vi "SQLGetDiagRec.vi"(4 "error in (no error)":errorcluster, 5 "HandleType":T1(ring)=enum."SQL_HANDLE_ENV", 6 "Status (SQL_SUCCESS=0)":i16, 7 "Input Handle":i32) -> (0 "error out":errorcluster, 3 "Output Handle":i32)   [LabVIEW 2011]
uses:
  Odbc32.dll
panel:
  in  "Boolean":bool
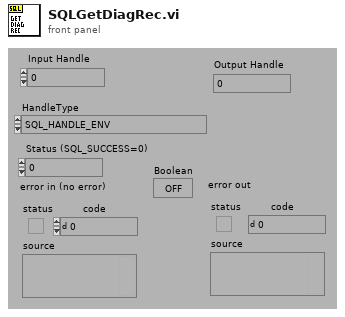
[diagram p1: front panel]
types:
  T1 = enum16{"NOPE", "SQL_HANDLE_ENV", "SQL_HANDLE_DBC", "SQL_HANDLE_STMT", "SQL_HANDLE_DESC"}
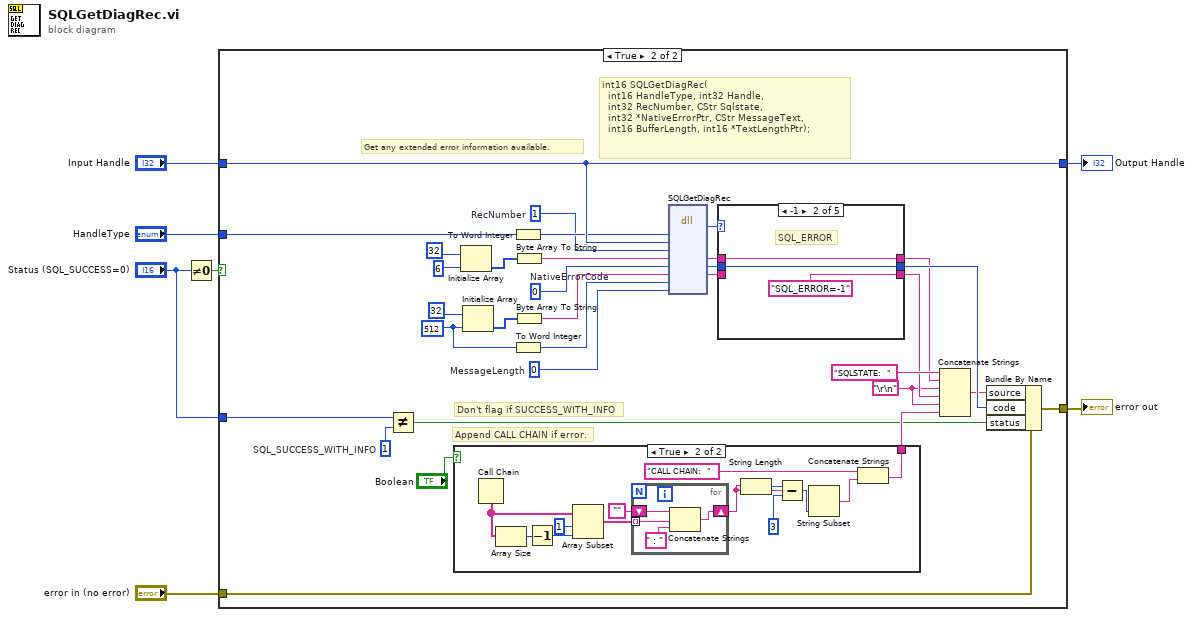
[diagram p0: block diagram]
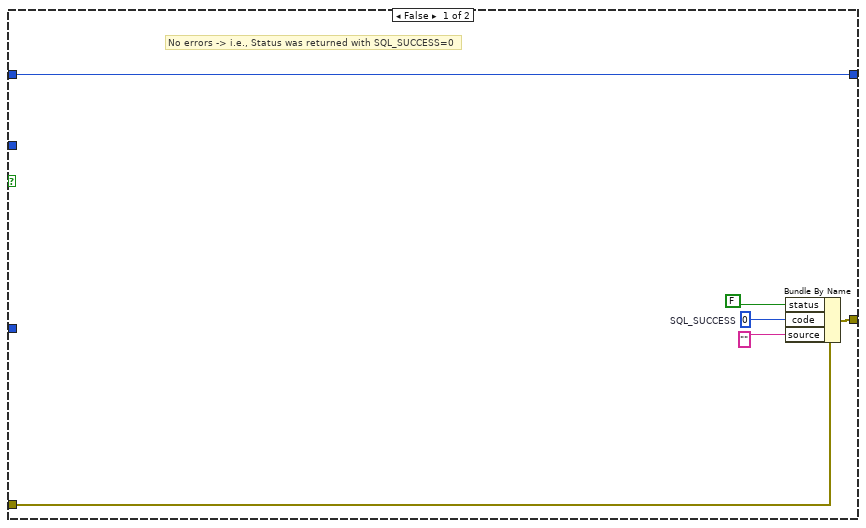
[diagram p2: hidden frame]
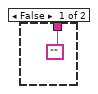
[diagram p3: hidden frame]
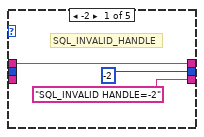
[diagram p4: hidden frame]
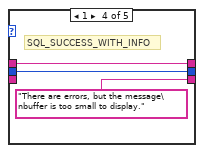
[diagram p6: hidden frame]
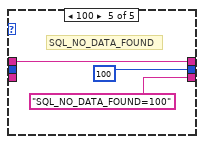
[diagram p7: hidden frame]
diagram:
  n1 = Not Equal To 0?(x="Status (SQL_SUCCESS=0)") -> (x != 0?=w7:bool)
  n2 = case shown="True" w7 {
    tunnel: "error in (no error)" -> [w12 w44]
    tunnel: [w11 w43] -> w1
    tunnel: [w13 w38] -> w4
    tunnel: "Input Handle" -> [w13 w38]
    tunnel: "HandleType" -> [_ w45]
    tunnel: "Status (SQL_SUCCESS=0)" -> [_ w42]
    frame False {
      w10 = 0  # SQL_SUCCESS
      # "No errors -> i.e., Status was returned with SQL_SUCCESS=0"
      n3 = Bundle By Name(cluster=w12, "status"=FALSE, "code"=w10, "source"="") -> (w11:errorcluster)
    }
    frame True {
      w26 = i16 0  # MessageLength
      w41 = i16 1  # SQL_SUCCESS_WITH_INFO
      w17 = "\r\n"
      w21 = 1  # RecNumber
      w28 = 512
      w32 = 0  # NativeErrorCode
      # "Append CALL CHAIN if error."
      # "Don't flag if SUCCESS_WITH_INFO"
      # "Get any extended error information available."
      # "int16 SQLGetDiagRec(\n  int16 HandleType, int32 Handle, \n  int32 RecNumber, CStr Sqlstate, \n  int32 *NativeErrorPtr, CStr MessageText, \n  int16 BufferLength, int16 *TextLengthPtr);"
      n4 = Not Equal?(x=w42, y=w41) -> (x != y?=w15:bool)
      n5 = case shown="True" "Boolean" {
        tunnel: ["" w48] -> w16
        frame False {
        }
        frame True {
          n6 = Call Chain() -> (call chain=w51:string[])
          n7 = Array Size(array=w51) -> (size(s)=w52:i32)
          n8 = Decrement(x=w52) -> (x-1=w47:i32)
          n9 = Array Subset(array=w51, index=1, length=w47) -> (w53:string[])
          n10 = for {
            tunnel: w53 -> [w62] mode=indexing
            shift-right: [w60] -> w55
            shift-left: "" -> [w61]
            n11 = Concatenate Strings(w61, w62, " : ") -> (w60:string)
          }
          n12 = String Length(string=w55) -> (length=w56:i32)
          n13 = Subtract(x=w56, y=3) -> (x-y=w57:i32)
          n14 = String Subset(string=w55, length (rest)=w57) -> (substring=w59:string)  [unwired: 1 out]
          n15 = Concatenate Strings("CALL CHAIN:  ", w59) -> (w48:string)
        }
      }
      n16 = Initialize Array(u8 32, 6) -> (w34:u8[])
      n17 = Initialize Array(u8 32, w28) -> (w30:u8[])
      n18 = To Word Integer(number=w45) -> (16bit integer=w37:i16)
      n19 = To Word Integer(number=w28) -> (16bit integer=w27:i16)
      n20 = Byte Array To String(unsigned byte array=w34) -> (string=w33:string)
      n21 = Byte Array To String(unsigned byte array=w30) -> (string=w29:string)
      n22 = dll-call lib="Odbc32.dll" fn="SQLGetDiagRec"("HandleType"=w37, "Handle"=w38, "RecNumber"=w21, "Sqlstate"=w33, "NativeErrorPtr"=w32, "MessageText"=w29, "BufferLength"=w27, "TextLengthPtr"=w26) -> ("Status"=w25:i16, "Sqlstate"=w24:string, "NativeErrorPtr"=w22:i32, "MessageText"=w23:string)  [unwired: 7 in, 3 out]
      n23 = case shown="-1" w25 {
        tunnel: [w66 w69 w72 w75 w78] -> w19
        tunnel: w24 -> [w66 w69 w72 w75 w78]
        tunnel: ["SQL_INVALID HANDLE=-2" "SQL_ERROR=-1" w70 "There are errors, but the message\nbuffer is too small to display." "SQL_NO_DATA_FOUND=100"] -> w18
        tunnel: w23 -> [_ _ w70 _ _]
        tunnel: [-2 w68 w71 w74 100] -> w40
        tunnel: w22 -> [_ w68 w71 w74 _]
        frame -2 {
          # "SQL_INVALID_HANDLE"
        }
        frame -1 {
          # "SQL_ERROR"
        }
        frame 0, Default {
          # "SQL_SUCCESS"
        }
        frame 1 {
          # "SQL_SUCCESS_WITH_INFO"
        }
        frame 100 {
          # "SQL_NO_DATA_FOUND"
        }
      }
      n24 = Concatenate Strings("SQLSTATE:  ", w19, w17, w18, w17, w16) -> (w39:string)
      n25 = Bundle By Name(cluster=w44, "source"=w39, "code"=w40, "status"=w15) -> (w43:errorcluster)
    }
  }
  "error out" <- w1
  "Output Handle" <- w4
